vi "snap_action.vi"(0 "HGF_ImaqUsb":refnum<class "HGF_ImaqUsb.lvclass">, 2 "Image In":T1, 5 "error in (no error)":errorcluster, 6 "Region of Interest":i32[](array[numeric]), 7 "Step x":i32=-1, 8 "Channel":i32=-1, 9 "Step y":i32=-1) -> (14 "dup HGF_ImaqUsb":refnum<class "HGF_ImaqUsb.lvclass">, 16 "Image Out":T1, 19 "error out":errorcluster)   [LabVIEW 2009, in "HGF_ImaqUsb.lvclass"]
doc: "Acquires a single image into <B>Image out</B>. A snap is appropriate for low-speed or single-capture applications where ease of programming is essential."
uses:
  HGF_ImaqUsb.lvclass
  <vilib>/vision/Image Controls.llb/IMAQ Image.ctl
  HGF_ImaqUsb.lvclass/HGF_ImaqUsb.ctl
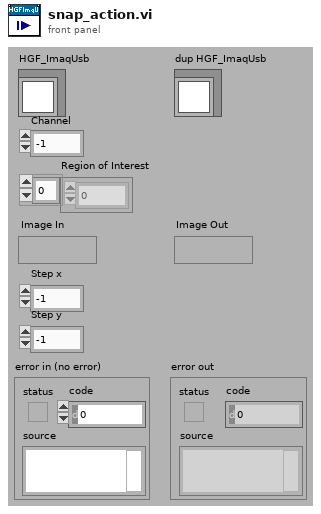
[diagram p1: front panel]
types:
  T1 = typedef "IMAQ Image.ctl" = refnum<image>
  T2 = typedef "IMAQ USB.ctl" = refnum<k1>
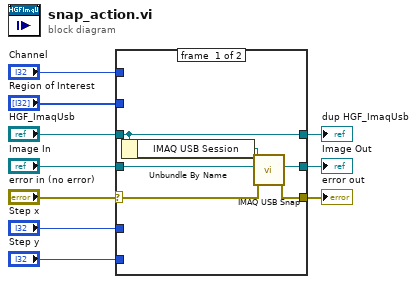
[diagram p0: block diagram]
diagram:
  n1 = case shown="No Error" "error in (no error)" {
    selector: "error in (no error)" -> [w14 w18]
    tunnel: "HGF_ImaqUsb" -> [w16 w17]
    tunnel: "Image In" -> [w13 w19]
    tunnel: "Region of Interest" -> [_ _]
    tunnel: "Step x" -> [_ _]
    tunnel: "Channel" -> [_ _]
    tunnel: "Step y" -> [_ _]
    tunnel: [w12 w19] -> w4
    tunnel: [w16 w17] -> w3
    tunnel: [w15 w18] -> w1
    frame #0 {
      n2 = Unbundle By Name(w16) -> ("IMAQ USB Session"=w11:T2)
      n3 = call <vilib>:"IMAQ USB Snap.vi"("error in (no error)"=w14, "Image in"=w13, "IMAQ USB Session In"=w11) -> ("error out"=w15:errorcluster, "Image out"=w12:T1)  [unwired: 7 out]
    }
    frame #1 {
    }
  }
  "error out" <- w1
  "dup HGF_ImaqUsb" <- w3
  "Image Out" <- w4
